vi "超标留样启动流程.vi"   [LabVIEW 2016, in "DR803M4.lvlib"]
uses:
  DR803M4.lvlib
  Global variable/input variable.vi
types:
  T1 = cluster{"远程留样":u16, "门禁标志":u16, "门禁密码":u32, "采样器进程":u16, "版本号":string, "启停":u16, "当前瓶号":u16, "采样模式选择":u16, "单次采样量":u16, "时间间隔":u16}
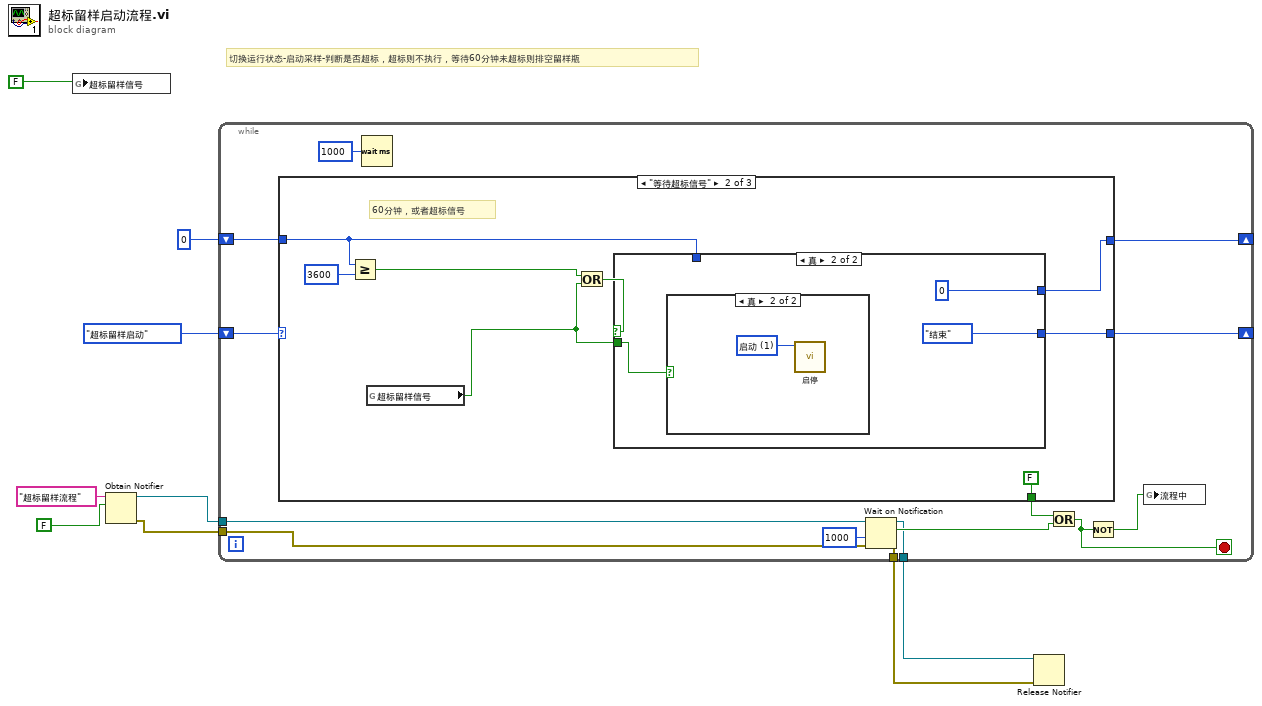
[diagram p0: block diagram]
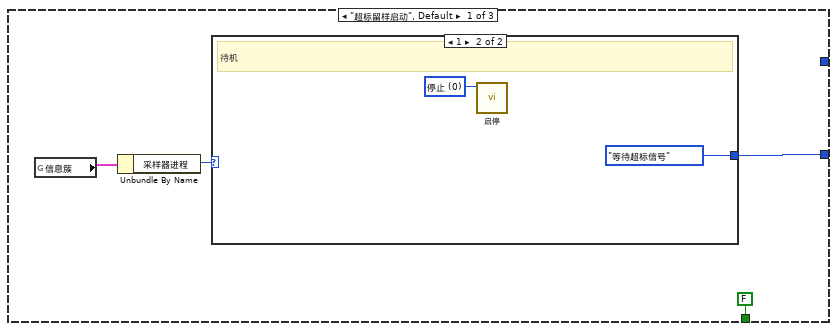
[diagram p2: hidden frame]
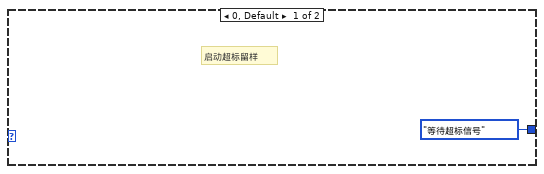
[diagram p3: hidden frame]
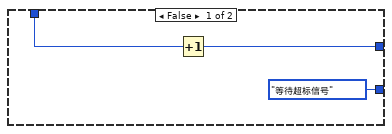
[diagram p4: hidden frame]
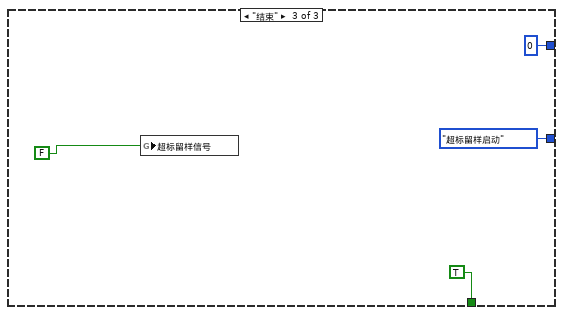
[diagram p6: hidden frame]
diagram:
  # "切换运行状态-启动采样-判断是否超标，超标则不执行，等待60分钟未超标则排空留样瓶"
  n1 = global write "input variable.vi" "超标留样信号"(FALSE ("采样完成")) -> ()
  n2 = Obtain Notifier(name (unnamed)="超标留样流程" ("名称（未命名）"), notification data type=FALSE ("采样完成")) -> (notifier out=w5:refnum<notifier>, error out=w4:errorcluster)  [unwired: 2 in, 1 out]
  n3 = while {
    shift-right: [w14] -> _
    shift-left: enum16{"超标留样启动", "等待超标信号", "结束"}."超标留样启动" -> [w23]
    shift-right: [w20] -> _
    shift-left: 0 -> [w21]
    tunnel: w5 -> [w19]
    tunnel: w4 -> [w18]
    tunnel: [w11] -> w2
    tunnel: [w10] -> w1
    stop <- w16 stop-if-true
    n4 = case shown="\"等待超标信号\"" w23 {
      tunnel: w21 -> [_ w34 _]
      tunnel: [_ w36 0] -> w20
      tunnel: [w25 w33 enum16{"超标留样启动", "等待超标信号", "结束"}."超标留样启动"] -> w14
      tunnel: [FALSE FALSE TRUE] -> w13
      frame "超标留样启动", Default {
        n5 = global read "input variable.vi" "信息簇"() -> (w27:T1)
        n6 = Unbundle By Name(w27) -> ("采样器进程"=w26:u16)
        n7 = case shown="1" w26 {
          tunnel: [enum16{"超标留样启动", "等待超标信号", "结束"}."等待超标信号" enum16{"超标留样启动", "等待超标信号", "结束"}."等待超标信号"] -> w25
          frame 0, Default {
            # "启动超标留样"
          }
          frame 1 {
            w29 = u16 0 items=["停止", "启动"] ("启停")
            # "待机"
            n8 = call "启停.vi"("启停"=w29) -> ()  [unwired: 10 in, 1 out]
          }
        }
      }
      frame "等待超标信号" {
        # "60分钟，或者超标信号"
        n9 = Greater Or Equal?(x=w34, y=3600) -> (x >= y?=w37:bool)
        n10 = global read "input variable.vi" "超标留样信号"() -> (w31:bool)
        n11 = Or(x=w37, y=w31) -> (x .or. y?=w35:bool)
        n12 = case shown="真" w35 {
          tunnel: [enum16{"超标留样启动", "等待超标信号", "结束"}."等待超标信号" enum16{"超标留样启动", "等待超标信号", "结束"}."结束"] -> w33
          tunnel: w34 -> [w41 _]
          tunnel: [w40 0] -> w36
          tunnel: w31 -> [_ w42]
          frame False {
            n13 = Increment(x=w41) -> (x+1=w40:i32)
          }
          frame True {
            n14 = case shown="真" w42 {
              frame False {
              }
              frame True {
                w45 = u16 1 items=["停止", "启动"] ("启停")
                n15 = call "启停.vi"("启停"=w45) -> ()  [unwired: 10 in, 1 out]
              }
            }
          }
        }
      }
      frame "结束" {
        n16 = global write "input variable.vi" "超标留样信号"(FALSE ("采样完成")) -> ()
      }
    }
    n17 = Wait (ms)(milliseconds to wait=u32 1000 ("等待时间（毫秒）")) -> ()  [unwired: 1 out]
    n18 = Wait on Notification(notifier=w19, timeout in ms (-1)=1000 ("超时毫秒(-1)"), error in (no error)=w18) -> (notifier out=w11:refnum<notifier>, notification=w15:bool, error out=w10:errorcluster)  [unwired: 1 in, 1 out]
    n19 = Or(x=w13, y=w15) -> (x .or. y?=w16:bool)
    n20 = Not(x=w16) -> (.not. x?=w12:bool)
    n21 = global write "input variable.vi" "流程中"(w12) -> ()
  }
  n22 = Release Notifier(notifier=w2, error in (no error)=w1) -> ()  [unwired: 1 in, 3 out]
